vi "Carbide-Get-AttValue.vi"(8 "Error In":errorcluster) -> (0 "Error Out":errorcluster, 3 "value":dbl)   [LabVIEW 2014]
doc: "André Romero - 2021\nandretec@ifsc.usp.br\nIFSC - USP"
uses:
  Carbide-Global.vi
  <vilib>/httpClient/LabVIEWHTTPClient.lvlib
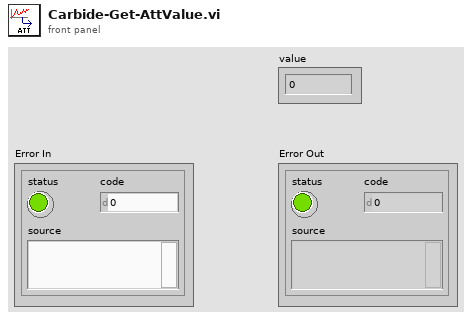
[diagram p1: front panel]
types:
  T1 = typedef "LabVIEWHTTPClient.lvlib/ClientHandle.ctl" = refnum<k1>
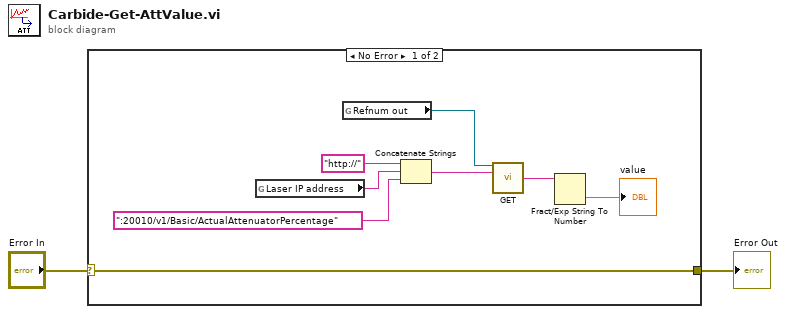
[diagram p0: block diagram]
diagram:
  n1 = case shown="No Error" "Error In" {
    selector: "Error In" -> [w3 w11]
    tunnel: [w3 w11] -> w1
    frame No Error {
      n2 = global read "Carbide-Global.vi" "Laser IP address"() -> (w7:string)
      n3 = global read "Carbide-Global.vi" "Refnum out"() -> (w10:T1)
      n4 = Concatenate Strings("http://" ("string"), w7, ":20010/v1/Basic/ActualAttenuatorPercentage" ("string")) -> (w9:string)
      n5 = call <vilib>:"GET.vi"("client handle"=w10, "url"=w9) -> ("body"=w5:string)  [unwired: 10 in, 3 out]
      n6 = Fract/Exp String To Number(string=w5) -> (number=→"value":dbl)  [unwired: 3 in, 1 out]
    }
    frame Error {
    }
  }
  "Error Out" <- w1
